vi "getData.vi"(8 "error in (no error)":errorcluster, 10 "Game":refnum<class "Game.lvclass">, 11 "Communication in":refnum<class "Communication.lvclass">) -> (0 "error out":errorcluster, 1 "Total Delay":dbl format="%#.5g", 2 "Robot Data":T1[](array[typedef]), 3 "Communication out":refnum<class "Communication.lvclass">, 4 "Team Color":enum16{"Azul", "Amarelo"}(ring), 5 "AllyRef":refnum<class "Ally.lvclass">)   [LabVIEW 2018, in "Communication.lvclass"]
uses:
  Communication.lvclass
  Game_class/Game.lvclass
  Paths/Convert AI Robot to Robot Command Folder/grSim/grSim Robot Command.ctl
  Ally_class/Ally.lvclass
  C:/Users/anton/Desktop/roboime/dar push/SSL_AI/SSL_AI/Team_class/Team.lvclass
  Game_class/Game.lvclass/Game.ctl
  Team_class/Team.lvclass/Team.ctl
  Robot_class/Robot.lvclass/Robot.ctl
  Robot_class/Read id.vi
  Robot_class/Read kick_x.vi
  Robot_class/Read kick_z.vi
  Robot_class/Read v_tang.vi
  Robot_class/Read v_norm.vi
  Robot_class/Read v_ang.vi
  Robot_class/Read dribble.vi
  Game_class/Read AllyRef.vi
  Game_class/Read TimeRef.vi
  Game_class/Read KeeperTeam.vi
  Game_class/Read OffensiveTeam.vi
  Game_class/Read DefensiveTeam.vi
  Game_class/Read NavigationTeam.vi
  Team_class/Read RobotRef.vi
  Team_class/Write RobotRef.vi
  Robot_class/Robot.lvclass
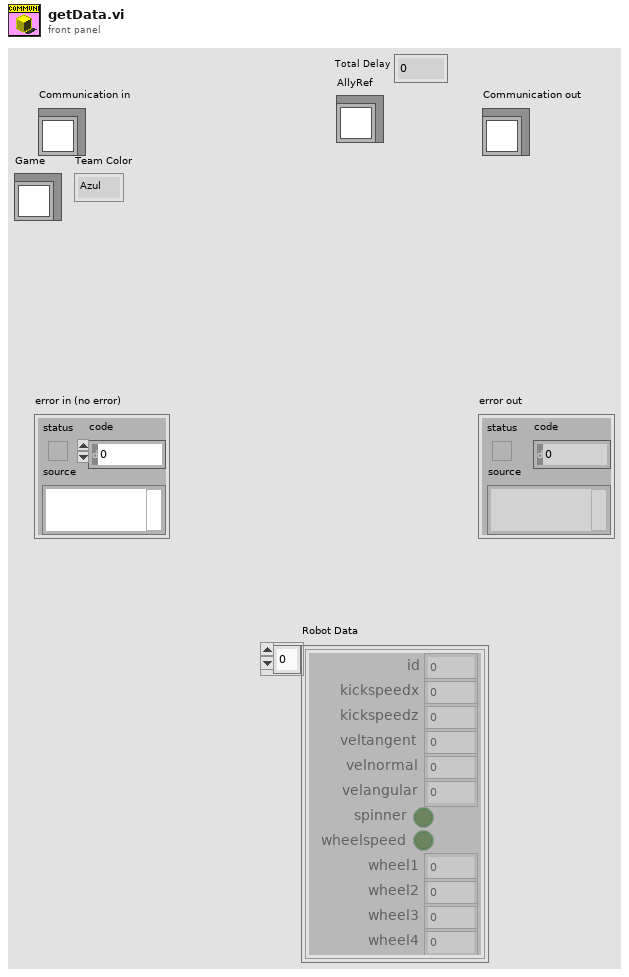
[diagram p1: front panel]
types:
  T1 = typedef "grSim Robot Command.ctl" = cluster{"id":u32, "kickspeedx":sgl, "kickspeedz":sgl, "veltangent":sgl, "velnormal":sgl, "velangular":sgl, "spinner":bool, "wheelspeed":bool, "wheel1":sgl, "wheel2":sgl, "wheel3":sgl, "wheel4":sgl}
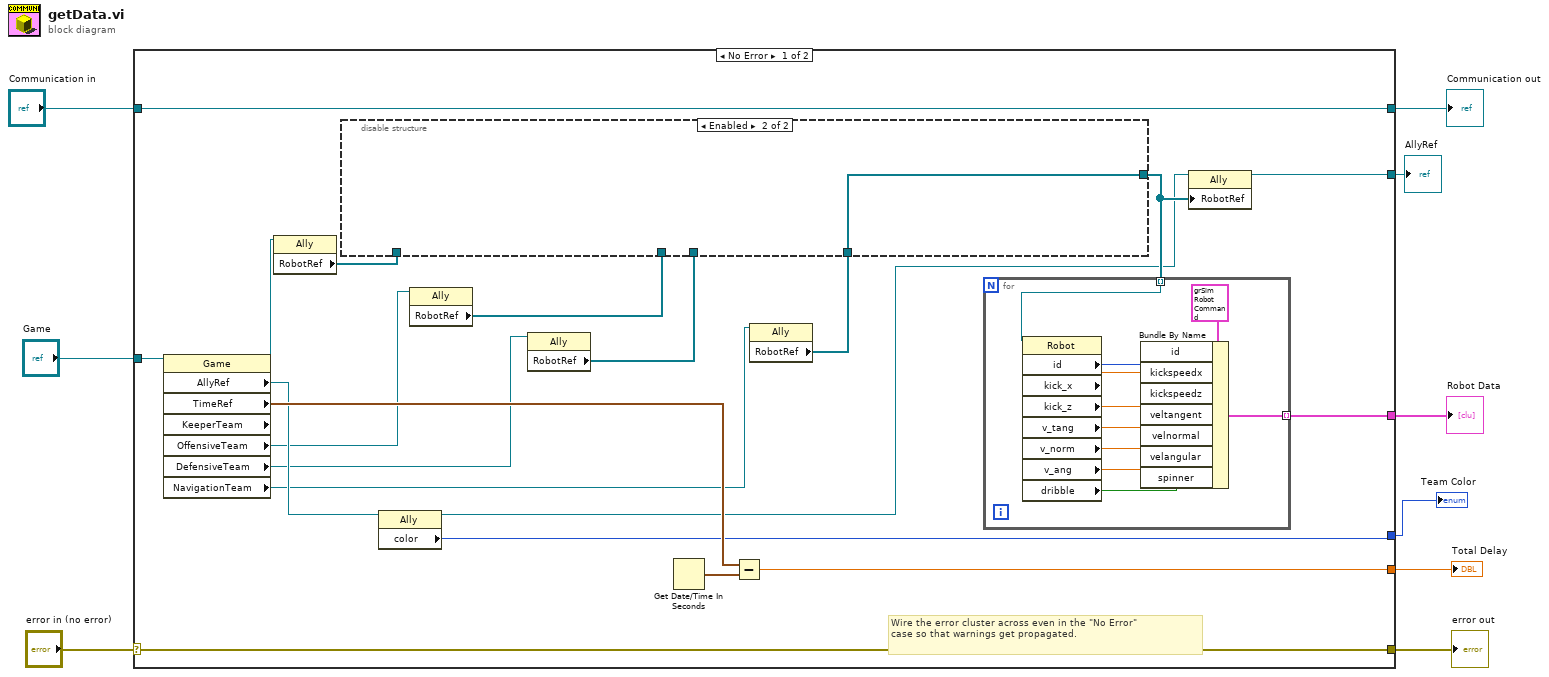
[diagram p0: block diagram]
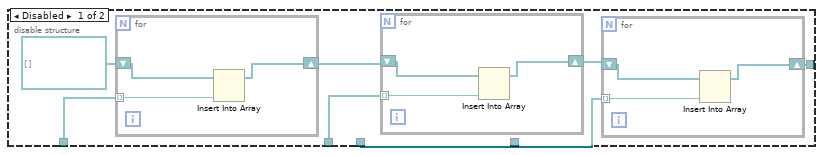
[diagram p2: hidden frame]
diagram:
  n1 = case shown="No Error" "error in (no error)" {
    selector: "error in (no error)" -> [w28 w58]
    tunnel: [w28 w58] -> w8
    tunnel: [w29 w57] -> w6
    tunnel: "Communication in" -> [w29 w57]
    tunnel: "Game" -> [w27 _]
    tunnel: [w25 _] -> w4
    tunnel: [w22 _] -> w3
    tunnel: [w21 _] -> w2
    tunnel: [w13 _] -> w1
    frame No Error {
      # "Wire the error cluster across even in the \"No Error\"\ncase so that warnings get propagated."
      n2 = property class="Game"(reference=w27) -> ("AllyRef"=w23:refnum<class "Ally.lvclass">, "TimeRef"=w26:timestamp, "KeeperTeam"=w20:refnum<class "Ally.lvclass">, "OffensiveTeam"=w18:refnum<class "Ally.lvclass">, "DefensiveTeam"=w16:refnum<class "Ally.lvclass">, "NavigationTeam"=w11:refnum<class "Ally.lvclass">)  [unwired: 1 in, 2 out]
      n3 = property class="Ally"(reference=w20) -> ("RobotRef"=w19:refnum<class "Robot.lvclass">[])  [unwired: 1 in, 2 out]
      n4 = property class="Ally"(reference=w23) -> (reference out=w12:refnum<class "Ally.lvclass">, "color"=w21:enum16{"Azul", "Amarelo"})  [unwired: 1 in, 1 out]
      n5 = property class="Ally"(reference=w18) -> ("RobotRef"=w17:refnum<class "Robot.lvclass">[])  [unwired: 1 in, 2 out]
      n6 = property class="Ally"(reference=w16) -> ("RobotRef"=w15:refnum<class "Robot.lvclass">[])  [unwired: 1 in, 2 out]
      n7 = Get Date/Time In Seconds() -> (seconds since 1Jan1904=w24:timestamp)
      n8 = Subtract(x=w26, y=w24) -> (x-y=w25:dbl)
      n9 = property class="Ally"(reference=w11) -> ("RobotRef"=w10:refnum<class "Robot.lvclass">[])  [unwired: 1 in, 2 out]
      n10 = disable-structure shown="Enabled" {
        disable-tunnel: w19 -> [w36 _]
        disable-tunnel: w17 -> [w34 _]
        disable-tunnel: w15 -> [w31 _]
        disable-tunnel: [w30 w46] -> w14
        disable-tunnel: w10 -> [_ w46]
        frame Disabled {
          n11 = for {
            tunnel: w36 -> [w43] mode=indexing
            shift-right: [w45] -> w33
            shift-left: refnum<class "Robot.lvclass">[] [] -> [w44]
            n12 = Insert Into Array(array=w44, new element=w43) -> (w45:refnum<class "Robot.lvclass">[])  [unwired: 1 in]
          }
          n13 = for {
            tunnel: w34 -> [w40] mode=indexing
            shift-right: [w42] -> w32
            shift-left: w33 -> [w41]
            n14 = Insert Into Array(array=w41, new element=w40) -> (w42:refnum<class "Robot.lvclass">[])  [unwired: 1 in]
          }
          n15 = for {
            tunnel: w31 -> [w37] mode=indexing
            shift-right: [w39] -> w30
            shift-left: w32 -> [w38]
            n16 = Insert Into Array(array=w38, new element=w37) -> (w39:refnum<class "Robot.lvclass">[])  [unwired: 1 in]
          }
        }
        frame Enabled {
        }
      }
      n17 = for {
        tunnel: [w48] -> w22 mode=indexing
        tunnel: w14 -> [w47] mode=indexing
        n18 = property class="Robot"(reference=w47) -> ("id"=w55:i32, "kick_x"=w54:dbl, "kick_z"=w53:dbl, "v_tang"=w52:dbl, "v_norm"=w51:dbl, "v_ang"=w50:dbl, "dribble"=w49:bool)  [unwired: 1 in, 2 out]
        n19 = Bundle By Name(cluster=T1 {"id"=0, "kickspeedx"=0.0, "kickspeedz"=0.0, "veltangent"=0.0, "velnormal"=0.0, "velangular"=0.0, "spinner"=FALSE, "wheelspeed"=FALSE, "wheel1"=0.0, "wheel2"=0.0, "wheel3"=0.0, "wheel4"=0.0} ("grSim Robot Command"), "id"=w55, "kickspeedx"=w54, "kickspeedz"=w53, "veltangent"=w52, "velnormal"=w51, "velangular"=w50, "spinner"=w49) -> (w48:T1)
      }
      n20 = property class="Ally"(reference=w12, "RobotRef"=w14) -> (reference out=w13:refnum<class "Ally.lvclass">)  [unwired: 1 in, 1 out]
    }
    frame Error {
    }
  }
  "error out" <- w8
  "Communication out" <- w6
  "Total Delay" <- w4
  "Robot Data" <- w3
  "Team Color" <- w2
  "AllyRef" <- w1
